vi "_Parse Detected Allocation List.vi"(8 "error in (no error)":errorcluster, 10 "Input String":string, 11 "VISA resource name":refnum<visa-resource-name>) -> (0 "error out":errorcluster, 1 "Detected Allocations":T1(array[cluster]), 2 "Reliability":i32, 3 "VISA resource name out":refnum<visa-resource-name>)   [LabVIEW 2020, in "Rohde&Schwarz CMWXP NR FR1 Measurement.lvlib"]
uses:
  <instrlib>/Rohde&Schwarz CMWXP NR FR1 Measurement/Rohde&Schwarz CMWXP NR FR1 Measurement.lvlib
  <instrlib>/Rohde&Schwarz CMWXP NR FR1 Measurement/Private/rsidr_core.llb/rsidr_core.lvlib
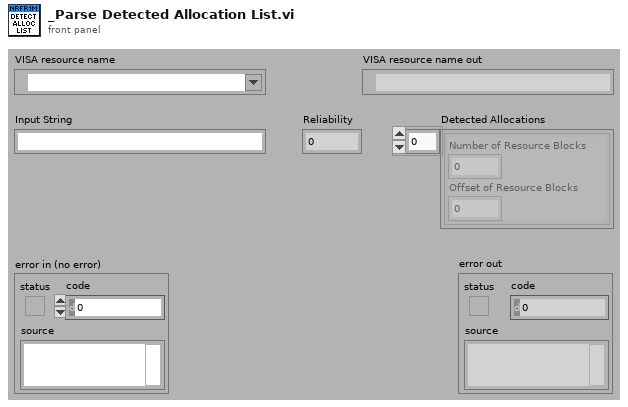
[diagram p1: front panel]
types:
  T1 = cluster{"Number of Resource Blocks":i32, "Offset of Resource Blocks":i32}[]
  T2 = cluster{"Nr Res Blocks":i32, "Offset Res Blocks":i32}
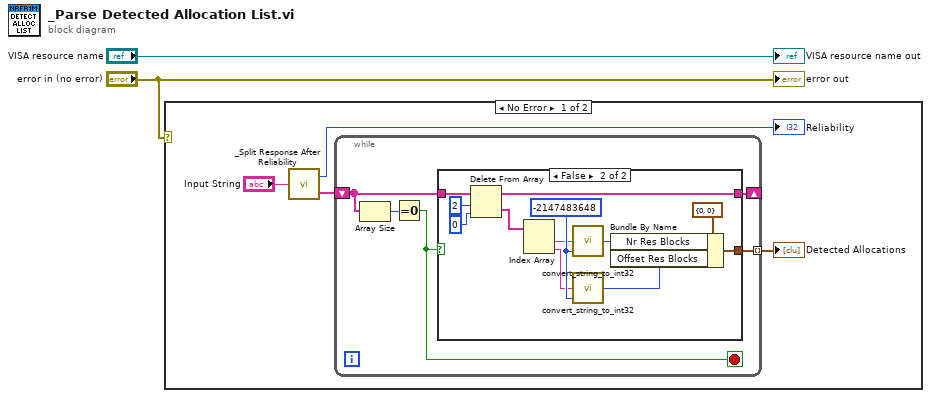
[diagram p0: block diagram]
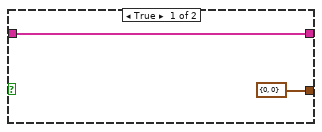
[diagram p2: hidden frame]
diagram:
  n1 = case shown="No Error" "error in (no error)" {
    frame No Error {
      n2 = call <instrlib>:"_Split Response After Reliability.vi"("Input String"="Input String") -> ("Response out"=w3:string[], "Reliability out"=→"Reliability":i32)
      n3 = while {
        tunnel: [w11] -> w4 mode=indexing
        shift-right: [w8] -> _
        shift-left: w3 -> [w10]
        stop <- w7 stop-if-true
        n4 = Array Size(array=w10) -> (size(s)=w9:i32)
        n5 = Equal To 0?(x=w9) -> (x = 0?=w7:bool)
        n6 = case shown="False" w7 {
          tunnel: [T2 {"Nr Res Blocks"=0, "Offset Res Blocks"=0} ("Detected Allocation") w23] -> w11
          tunnel: w10 -> [w12 w18]
          tunnel: [w12 w17] -> w8
          frame True {
          }
          frame False {
            w25 = -2147483648
            n7 = Delete From Array(array=w18, length=2, index=0) -> (deleted portion=w14:string[], array with subset deleted=w17:string[])
            n8 = Index Array(array=w14) -> (element #1=w20:string, element #2=w19:string)  [unwired: 2 in]
            n9 = call <instrlib>:"convert_string_to_int32.vi"("default (0)"=w25, "String in"=w20) -> ("int32 value out"=w22:i32)  [unwired: 3 in]
            n10 = call <instrlib>:"convert_string_to_int32.vi"("default (0)"=w25, "String in"=w19) -> ("int32 value out"=w21:i32)  [unwired: 3 in]
            n11 = Bundle By Name(cluster=T2 {"Nr Res Blocks"=0, "Offset Res Blocks"=0} ("Detected Allocation"), "Nr Res Blocks"=w22, "Offset Res Blocks"=w21) -> (w23:T2)
          }
        }
      }
      "Detected Allocations" <- w4
    }
    frame Error {
    }
  }
  "VISA resource name out" <- "VISA resource name"
  "error out" <- "error in (no error)"
